vi "Waveform Cluster to Array.vi"(11 "Waveform Cluster":T1) -> (3 "Array":waveform(dbl)[](array[waveform]))   [LabVIEW 2023]
uses:
  controls/Waveforms.ctl
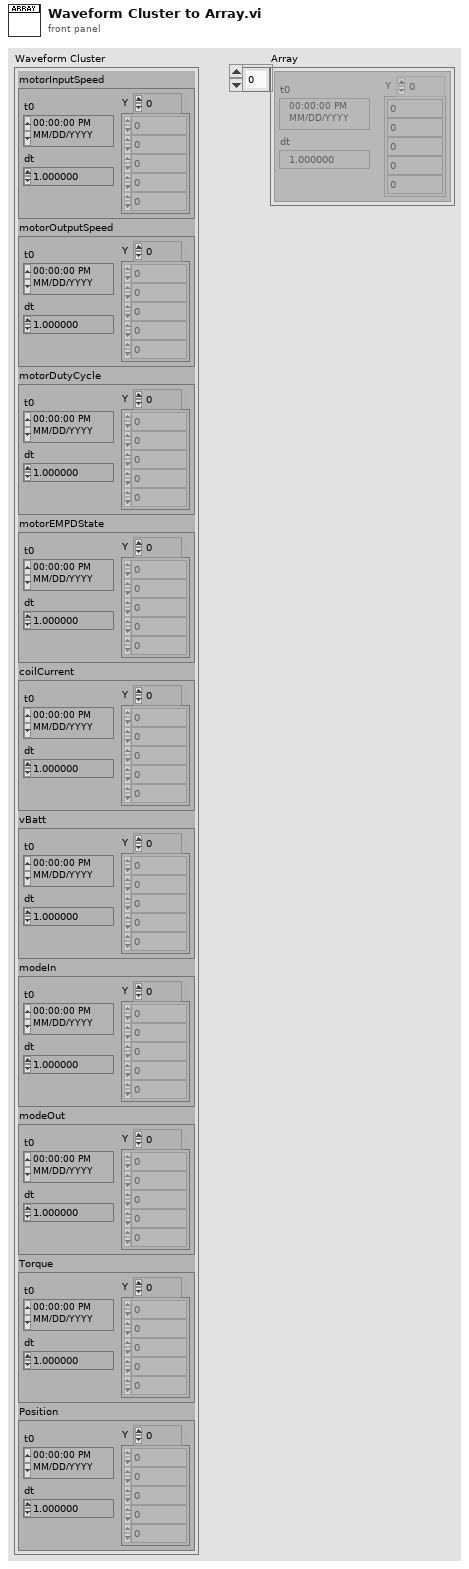
[diagram p1: front panel]
types:
  T1 = typedef "Waveforms.ctl" = cluster{"motorInputSpeed":waveform(dbl), "motorOutputSpeed":waveform(dbl), "motorDutyCycle":waveform(dbl), "motorEMPDState":waveform(dbl), "coilCurrent":waveform(dbl), "vBatt":waveform(dbl), "modeIn":waveform(dbl), "modeOut":waveform(dbl), "Torque":waveform(dbl), "Position":waveform(dbl)}
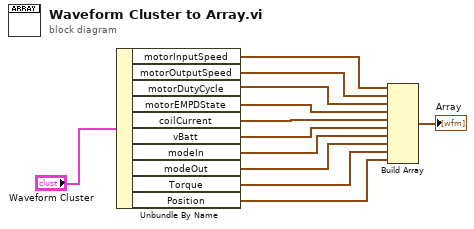
[diagram p0: block diagram]
diagram:
  n1 = Unbundle By Name("Waveform Cluster") -> ("motorInputSpeed"=w1:waveform(dbl), "motorOutputSpeed"=w2:waveform(dbl), "motorDutyCycle"=w4:waveform(dbl), "motorEMPDState"=w5:waveform(dbl), "coilCurrent"=w6:waveform(dbl), "vBatt"=w7:waveform(dbl), "modeIn"=w8:waveform(dbl), "modeOut"=w3:waveform(dbl), "Torque"=w11:waveform(dbl), "Position"=w12:waveform(dbl))
  n2 = Build Array(w1, w2, w4, w5, w6, w7, w8, w3, w11, w12) -> (→"Array":waveform(dbl)[])
